vi "Keithley 6487 Setup.vi"() -> (0 "error out":errorcluster, 1 "VISA resource name out":refnum<visa-resource-name>)   [LabVIEW 2020]
uses:
  <vilib>/Instr/_visa.llb/VISA Configure Serial Port (Instr).vi
panel:
  in  "Initial Configuration":string="*RST;:SYST:ZCH 1;:CURR:RANG 2E-9;:INIT;:SYST:ZCOR:ACQ;:SYST:ZCOR 1;:CURR:RANG:AUTO 1;:SYST:ZCH 0;"
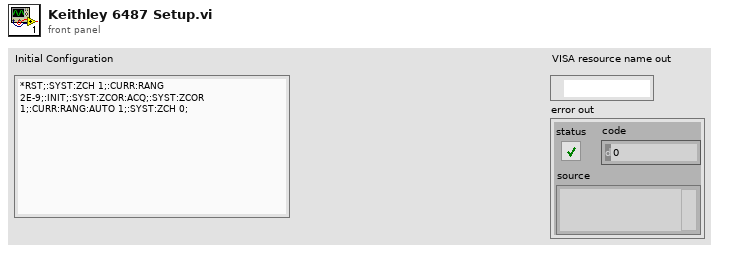
[diagram p1: front panel]
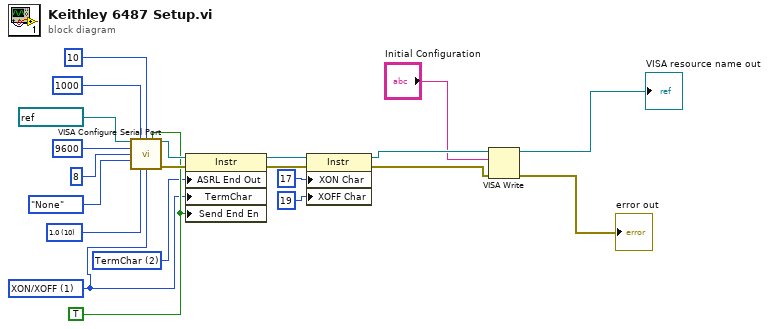
[diagram p0: block diagram]
diagram:
  w10 = u16 2 items=["None", "Last Bit", "TermChar", "Break"] ("Serial Settings:End Mode for Writes")
  w12 = TRUE ("Enable Termination\nChar (T)")
  w11 = u16 1 items=["None", "XON/XOFF", "RTS/CTS", "XON/XOFF & RTS/CTS", "DTR/DSR", "XON/XOFF & DTR/DSR"] ("flow control (0:none)")
  w21 = u16 10 items=["1.0"=10, "1.5"=15, "2.0"=20] ("stop bits (10: 1 bit)")
  n1 = call-poly "VISA Configure Serial Port"("VISA resource name"=refnum<visa-resource-name> "COM 6", "timeout (10sec)"=u32 1000, "termination char\n(0xA = '\\n' = LF)"=u8 10 ("termination char\n(0xA = '\\n' = LF)"), "Enable Termination\nChar (T)"=w12, "baud rate (9600)"=u32 9600, "data bits (8)"=u16 8, "parity (0:none)"=enum16{"None", "Odd", "Even", "Mark", "Space"}."None", "stop bits (10: 1 bit)"=w21, "flow control (0:none)"=w11) -> ("VISA resource name out"=w14:refnum<visa-resource-name>, "error out"=w13:errorcluster)  [unwired: 5 in]
  n2 = property class="Instr"(reference=w14, error in=w13, "ASRL End Out"=w10, "TermChar"=w11, "Send End En"=w12) -> (reference out=w9:refnum<visa-resource-name>, error out=w8:errorcluster)
  n3 = property class="Instr"(reference=w9, error in=w8, "XON Char"=u8 17 ("Serial Settings:Flow Control XON Character"), "XOFF Char"=u8 19 ("Serial Settings:Flow Control XOFF Character")) -> (reference out=w5:refnum<visa-resource-name>, error out=w4:errorcluster)
  n4 = VISA Write(VISA resource name=w5, write buffer="Initial Configuration", error in (no error)=w4) -> (VISA resource name out=→"VISA resource name out":refnum<visa-resource-name>, error out=→"error out":errorcluster)  [unwired: 1 out]
